vi "Initialize.vi"(8 "error in (no error)":errorcluster, 9 "Ethernet Config":T2, 10 "Comm Interface":T1, 11 "Device ID (0)":i32) -> (0 "error out":errorcluster, 3 "Device ID out":i32)   [LabVIEW 8.6, in "Keyence LJ-V7000.lvlib"]
doc: "Communication with the controller is established.\nThis VI has to be executed for a controller specified with <B>Device ID</B> prior to other VI only once."
uses:
  Keyence LJ-V7000.lvlib
  constant/Driver VI No.ctl
  Clusters/Ethernet Config.ctl
  constant/Comm Interface.ctl
panel:
  # "(c) 2012 KEYENCE CORPORATION.  ALL RIGHTS RESERVED."
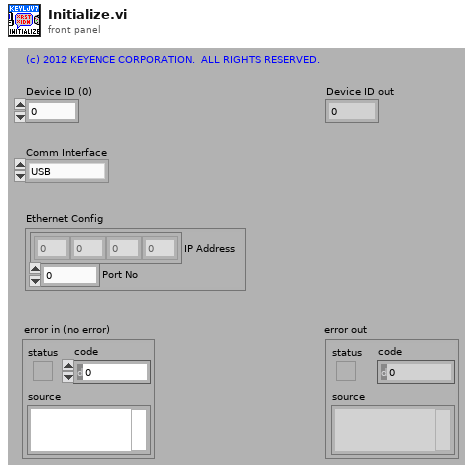
[diagram p1: front panel]
types:
  T1 = typedef "Keyence LJ-V7000.lvlib/Comm Interface.ctl" = enum8{"USB", "ETHERNET"}
  T2 = typedef "Keyence LJ-V7000.lvlib/Ethernet Config.ctl" = cluster{"IP Address":u8[], "Port No":u16}
  T3 = typedef "Keyence LJ-V7000.lvlib/Driver VI No.ctl" = enum16{"Initialize", "Close", "Reboot Controller", "Return to Factory State", "Get System Error", "Clear System Error", "Trigger", "Start Batch Measurements", "Stop Batch Measurements", "Auto Zero", "Timing", "Reset", "Clear Memory", "Set Setting", "Get Setting", "Initialize Setting", "Reflect Setting", "Update Write Settings Area", "Check Status of Saving to Save Area", "Set Time", "Get Time", "Change Program", "Read Active Program Number", "Read Measurement Data", "Read Profiles(for High-Speed Mode)", "Read Batch Profiles(for High-Speed Mode)", "Read Profiles(for Advanced Mode)", "Read Batch Profiles(for Advanced Mode)", "Start Storage", "Stop Storage", "Read Storage Status", "Read Data Storage Data", "Read Profile Storage Data", "Read Batch Profile Storage Data", "Start High-Speed Data Communication", "Stop High-Speed Data Communication", "Read Profiles(for High-Speed Communication)"}
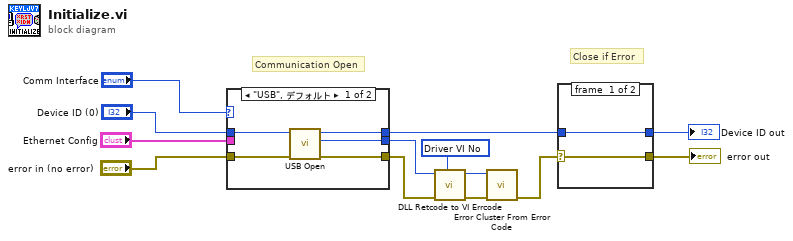
[diagram p0: block diagram]
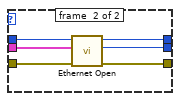
[diagram p2: hidden frame]
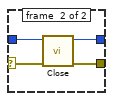
[diagram p3: hidden frame]
diagram:
  # "Close if Error"
  # "Communication Open"
  n1 = case shown="\"USB\", デフォルト" "Comm Interface" {
    tunnel: "Device ID (0)" -> [w18 w23]
    tunnel: "error in (no error)" -> [w17 w24]
    tunnel: "Ethernet Config" -> [_ w22]
    tunnel: [w15 w21] -> w4
    tunnel: [w16 w20] -> w7
    tunnel: [w14 w19] -> w6
    frame #0 {
      n2 = call "USB Open.vi"("error in (no error)"=w17, "Device ID"=w18) -> ("error out"=w15:errorcluster, "Return Code"=w14:i32, "Device ID out"=w16:i32)  [unwired: 7 in]
    }
    frame #1 {
      n3 = call "Ethernet Open.vi"("error in (no error)"=w24, "Ethernet Config"=w22, "Device ID"=w23) -> ("error out"=w21:errorcluster, "Return Code"=w19:i32, "Device ID out"=w20:i32)  [unwired: 6 in]
    }
  }
  n4 = call "DLL Retcode to VI Errcode.vi"("Driver VI No"=T3 ?, "error in (no error)"=w4, "DLL Return Code"=w6) -> ("error out"=w3:errorcluster, "VI Error Code"=w2:i32)  [unwired: 7 in]
  n5 = call <vilib>:"Error Cluster From Error Code.vi"("error in (no error)"=w3, "error code (0)"=w2) -> ("error out"=w1:errorcluster)  [unwired: 7 in]
  n6 = case shown="エラー" w1 {
    selector: w1 -> [w26 w29]
    tunnel: [w26 w30] -> w13
    tunnel: w7 -> [w25 w28]
    tunnel: [w25 w27] -> w8
    frame #0 {
    }
    frame #1 {
      n7 = call "Close.vi"("error in (no error)"=w29, "Device ID (0)"=w28) -> ("error out"=w30:errorcluster, "Device ID out"=w27:i32)  [unwired: 8 in]
    }
  }
  "error out" <- w13
  "Device ID out" <- w8
